vi "Acquire Data from Hardware.vi"(7 "error in (no error)":errorcluster, 10 "Hardware Configuration":T1) -> (0 "error out":errorcluster, 2 "Graph Data":waveform(dbl)[](array[waveform]))   [LabVIEW 2022 SP3]
doc: "Generates sample waveforms according to the signal type in the HW Config input."
uses:
  controls/HW Configuration.ctl
  controls/AccelerometerSettings.ctl
  <vilib>/DAQmx/read.llb/DAQmx Read (Analog 1D Wfm NChan NSamp).vi
  <vilib>/DAQmx/create/channels.llb/DAQmx Create Channel (AI-Acceleration-Accelerometer).vi
  <vilib>/DAQmx/configure/timing.llb/DAQmx Timing (Sample Clock).vi
  <vilib>/DAQmx/miscellaneous.llb/DAQmx Fill In Error Info.vi
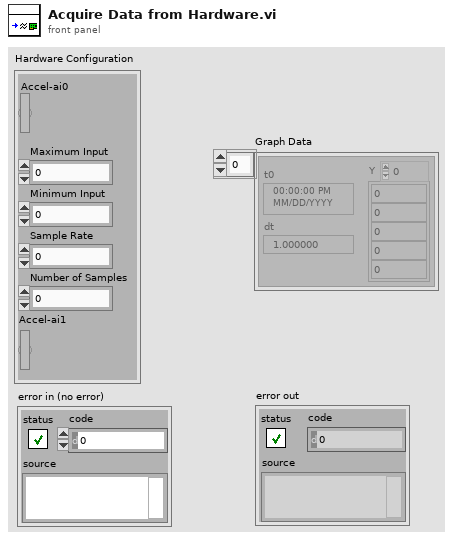
[diagram p1: front panel]
types:
  T1 = typedef "HW Configuration.ctl" = cluster{"Accel-ai0":bool, "Maximum Input":dbl, "Minimum Input":dbl, "Sample Rate":dbl, "Number of Samples":i32, "Accel-ai1":bool}
  T2 = typedef "AccelerometerSettings.ctl" = cluster{"current excitation source":i32, "current excitation value":dbl, "name to assign":string, "physical channels":tag, "sensitivity":dbl, "sensitivity units":i32, "units":i32}
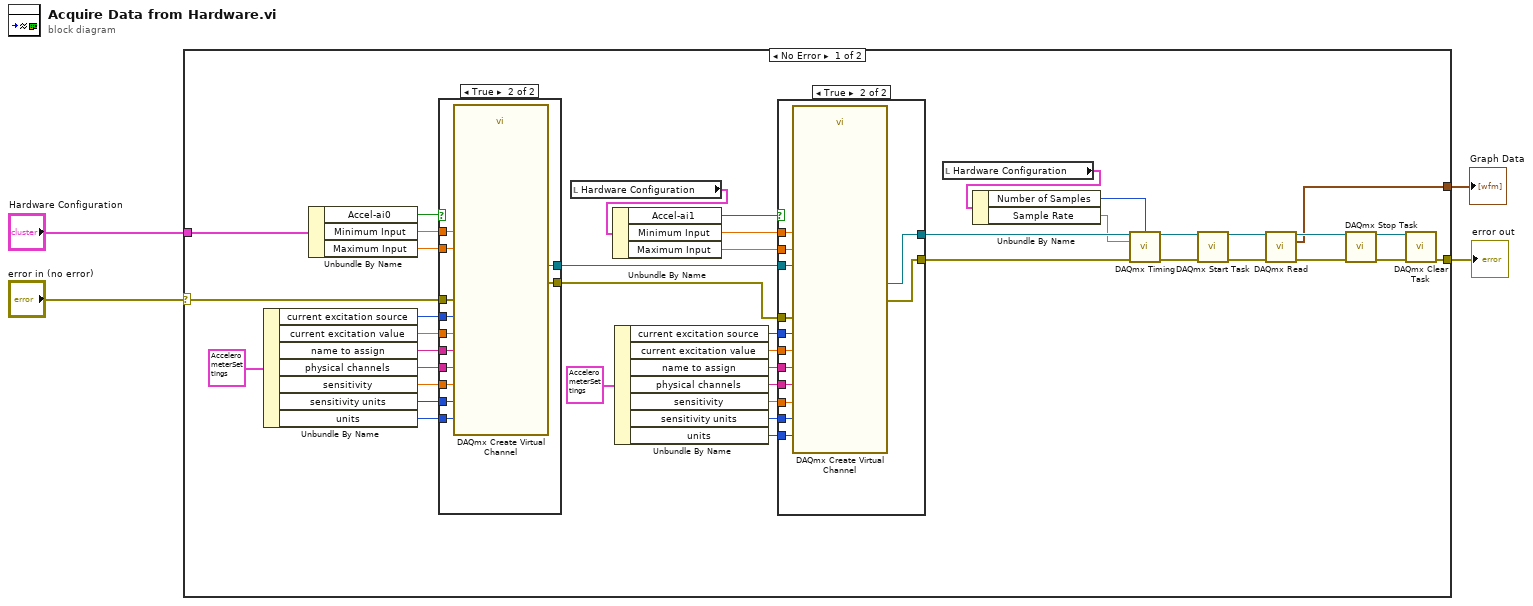
[diagram p0: block diagram]
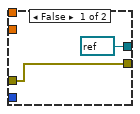
[diagram p3: hidden frame]
diagram:
  n1 = case shown="No Error" "error in (no error)" {
    selector: "error in (no error)" -> [w37 w76]
    tunnel: [w38 w76] -> w3
    tunnel: "Hardware Configuration" -> [w46 _]
    tunnel: [w41 _] -> w1
    frame No Error {
      n2 = Unbundle By Name(T2 {"current excitation source"=10200, "current excitation value"=0.002, "name to assign"="Accel-ai0", "physical channels"="NI-USB-4431/ai0", "sensitivity"=10.0, "sensitivity units"=12509, "units"=12470}) -> ("current excitation source"=w33:i32, "current excitation value"=w32:dbl, "name to assign"=w31:string, "physical channels"=w30:tag, "sensitivity"=w29:dbl, "sensitivity units"=w28:i32, "units"=w27:i32)
      n3 = Unbundle By Name(w46) -> ("Accel-ai0"=w8:bool, "Minimum Input"=w10:dbl, "Maximum Input"=w9:dbl)
      n4 = case shown="True" w8 {
        tunnel: w37 -> [w63 w75]
        tunnel: [w63 w74] -> w17
        tunnel: [refnum<k21> refnum ("task out") w73] -> w25
        tunnel: w33 -> [_ w72]
        tunnel: w32 -> [_ w71]
        tunnel: w31 -> [_ w70]
        tunnel: w30 -> [_ w69]
        tunnel: w29 -> [_ w68]
        tunnel: w28 -> [_ w67]
        tunnel: w27 -> [_ w66]
        tunnel: w10 -> [_ w65]
        tunnel: w9 -> [_ w64]
        frame False {
        }
        frame True {
          n5 = call-poly <vilib>:"DAQmx Create Virtual Channel.vi"("maximum value"=w64, "minimum value"=w65, "physical channels"=w69, "current excitation source"=w72, "name to assign"=w70, "current excitation value"=w71, "units"=w66, "error in"=w75, "sensitivity"=w68, "sensitivity units"=w67) -> ("task out"=w73:refnum<k21>, "error out"=w74:errorcluster)  [unwired: 4 in]
        }
      }
      n6 = local read "Hardware Configuration"() -> (w14:T1)
      n7 = Unbundle By Name(w14) -> ("Accel-ai1"=w11:bool, "Minimum Input"=w12:dbl, "Maximum Input"=w13:dbl)
      n8 = Unbundle By Name(T2 {"current excitation source"=10200, "current excitation value"=0.002, "name to assign"="Accel-ai1", "physical channels"="NI-USB-4431/ai1", "sensitivity"=10.0, "sensitivity units"=12509, "units"=12470}) -> ("current excitation source"=w18:i32, "current excitation value"=w19:dbl, "name to assign"=w20:string, "physical channels"=w21:tag, "sensitivity"=w22:dbl, "sensitivity units"=w23:i32, "units"=w24:i32)
      n9 = case shown="True" w11 {
        tunnel: [w48 w61] -> w15
        tunnel: w22 -> [_ w58]
        tunnel: w25 -> [w48 w60]
        tunnel: w24 -> [_ w53]
        tunnel: w23 -> [_ w59]
        tunnel: w21 -> [_ w57]
        tunnel: w20 -> [_ w56]
        tunnel: w19 -> [_ w55]
        tunnel: w18 -> [_ w54]
        tunnel: w17 -> [w47 w52]
        tunnel: [w47 w51] -> w16
        tunnel: w13 -> [_ w50]
        tunnel: w12 -> [_ w49]
        frame False {
        }
        frame True {
          n10 = call-poly <vilib>:"DAQmx Create Virtual Channel.vi"("task in"=w60, "maximum value"=w50, "minimum value"=w49, "physical channels"=w57, "current excitation source"=w54, "name to assign"=w56, "current excitation value"=w55, "units"=w53, "error in"=w52, "sensitivity"=w58, "sensitivity units"=w59) -> ("task out"=w61:refnum<k21>, "error out"=w51:errorcluster)  [unwired: 3 in]
        }
      }
      n11 = local read "Hardware Configuration"() -> (w7:T1)
      n12 = Unbundle By Name(w7) -> ("Number of Samples"=w5:i32, "Sample Rate"=w6:dbl)
      n13 = call-poly <vilib>:"DAQmx Timing.vi"("task/channels in"=w15, "samples per channel"=w5, "rate"=w6, "error in"=w16) -> ("task out"=w36:refnum<k21>, "error out"=w35:errorcluster)  [unwired: 10 in]
      n14 = call <vilib>:"DAQmx Start Task.vi"("task/channels in"=w36, "error in"=w35) -> ("task out"=w45:refnum<k21>, "error out"=w44:errorcluster)  [unwired: 12 in]
      n15 = call-poly <vilib>:"DAQmx Read.vi"("task/channels in"=w45, "error in"=w44) -> ("task out"=w42:refnum<k21>, "data"=w41:waveform(dbl)[], "error out"=w43:errorcluster)  [unwired: 11 in]
      n16 = call <vilib>:"DAQmx Stop Task.vi"("task/channels in"=w42, "error in"=w43) -> ("task out"=w39:refnum<k21>, "error out"=w40:errorcluster)  [unwired: 12 in]
      n17 = call <vilib>:"DAQmx Clear Task.vi"("task in"=w39, "error in"=w40) -> ("error out"=w38:errorcluster)  [unwired: 13 in]
    }
    frame Error {
    }
  }
  "error out" <- w3
  "Graph Data" <- w1
